vi "C8855-01_CalcuP.vi"(8 "MainD":T1 {"G_DIM" format="%.5f"}, 10 "MP":u32=100 caption="Measurment points" min=1 max=100000, 11 "GT":i32(ring)=4 caption="Gate Time" items=["50 us", "100 us", "200 us", "500 us", "1 ms", "2 ms", "5 ms", "10 ms", "20 ms", "50 ms", "100 ms", "200 ms", "500ms", "1 s", "2 s", "5 s", "10 s"]) -> (0 "MainDR":T1 {"G_DIM" format="%.5f"})   [LabVIEW 2017]
uses:
  C8855_MainD.ctl
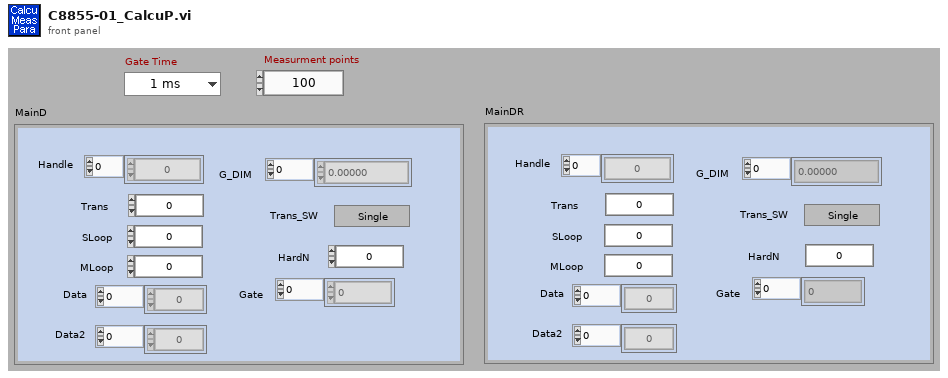
[diagram p1: front panel]
types:
  T1 = typedef "C8855_MainD.ctl" = cluster{"Handle":i64[], "G_DIM":dbl[], "Trans":u16, "Trans_SW":bool, "HardN":i32, "Gate":u8[], "Data":u32[], "Data2":u32[], "SLoop":i32, "MLoop":i32}
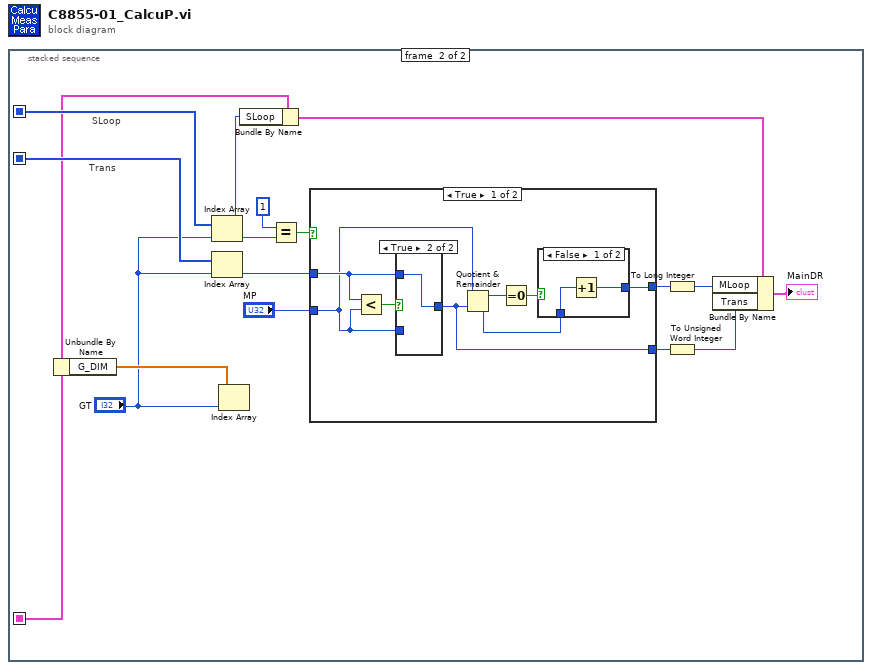
[diagram p0: block diagram]
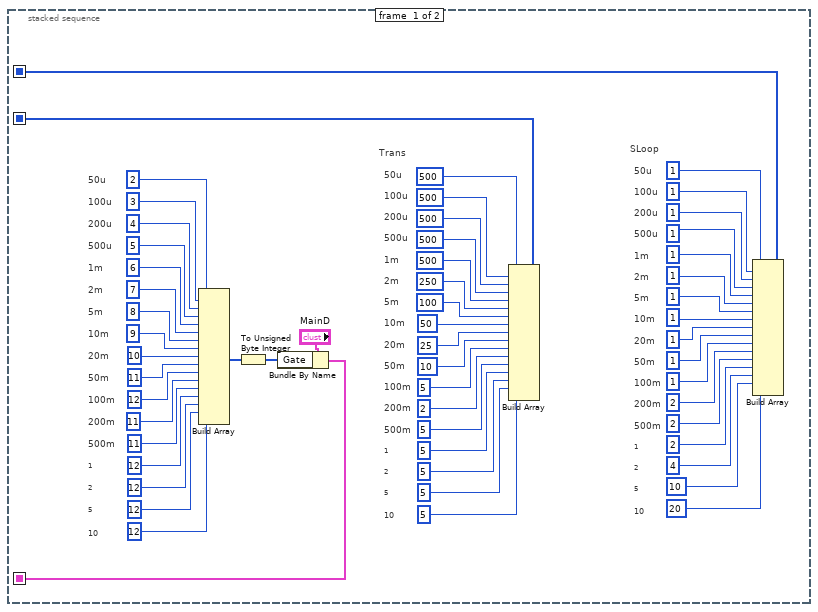
[diagram p2: hidden frame]
diagram:
  n1 = stacked-sequence {
    seq-local: [w1 _] -> [_ w63]
    seq-local: [w5 _] -> [_ w70]
    seq-local: [w4 _] -> [_ w71]
    frame #0 {
      # "10"
      # "5"
      # "2"
      # "1"
      # "500m"
      # "200m"
      # "100m"
      # "50m"
      # "20m"
      # "10m"
      # "5m"
      # "2m"
      # "1m"
      # "500u"
      # "200u"
      # "100u"
      # "50u"
      # "10"
      # "5"
      # "2"
      # "1"
      # "500m"
      # "200m"
      # "100m"
      # "50m"
      # "20m"
      # "10m"
      # "5m"
      # "2m"
      # "1m"
      # "500u"
      # "200u"
      # "100u"
      # "50u"
      # "SLoop"
      # "Trans"
      # "10"
      # "5"
      # "2"
      # "1"
      # "500m"
      # "200m"
      # "100m"
      # "50m"
      # "20m"
      # "10m"
      # "5m"
      # "2m"
      # "1m"
      # "500u"
      # "200u"
      # "100u"
      # "50u"
      n2 = Build Array(2, 3, 4, 5, 6, 7, 8, 9, 10, 11, 12, 11, 11, 12, 12, 12, 12) -> (w23:i32[])
      n3 = To Unsigned Byte Integer(number=w23) -> (unsigned 8bit integer=w2:u8[])
      n4 = Bundle By Name(cluster="MainD", "Gate"=w2) -> (w1:T1)
      n5 = Build Array(u16 500, u16 500, u16 500, u16 500, u16 500, u16 250, u16 100, u16 50, u16 25, u16 10, u16 5, u16 2, u16 5, u16 5, u16 5, u16 5, u16 5) -> (w5:u16[])
      n6 = Build Array(1 ("SLoop"), 1 ("SLoop"), 1 ("SLoop"), 1 ("SLoop"), 1 ("SLoop"), 1 ("SLoop"), 1 ("SLoop"), 1 ("SLoop"), 1 ("SLoop"), 1 ("SLoop"), 1 ("SLoop"), 2 ("SLoop"), 2 ("SLoop"), 2 ("SLoop"), 4 ("SLoop"), 10 ("SLoop"), 20 ("SLoop")) -> (w4:i32[])
    }
    frame #1 {
      # "Trans"
      # "SLoop"
      n7 = Unbundle By Name(w63) -> ("G_DIM"=w72:dbl[])
      n8 = Index Array(array=w71, index="GT") -> (element=w62:i32)
      n9 = Index Array(array=w70, index="GT") -> (element=w65:u16)
      n10 = Index Array(array=w72, index="GT") -> ()  [unwired: 1 out]
      n11 = Bundle By Name(cluster=w63, "SLoop"=w62) -> (w61:T1)
      n12 = Equal?(x=1, y=w62) -> (x = y?=w67:bool)
      n13 = case shown="True" w67 {
        tunnel: [w75 w88] -> w66
        tunnel: w65 -> [w80 w87]
        tunnel: "MP" -> [w79 w88]
        tunnel: [w74 w87] -> w59
        frame True {
          n14 = Less?(x=w80, y=w79) -> (x < y?=w81:bool)
          n15 = case shown="True" w81 {
            tunnel: w79 -> [w85 _]
            tunnel: w80 -> [_ w86]
            tunnel: [w85 w86] -> w74
            frame False {
            }
            frame True {
            }
          }
          n16 = Quotient & Remainder(x=w79, y=w74) -> (x-y*floor(x/y)=w78:u32, floor(x/y)=w76:u32)
          n17 = Equal To 0?(x=w78) -> (x = 0?=w77:bool)
          n18 = case shown="False" w77 {
            tunnel: w76 -> [w83 w84]
            tunnel: [w82 w84] -> w75
            frame False {
              n19 = Increment(x=w83) -> (x+1=w82:u32)
            }
            frame True {
            }
          }
        }
        frame False {
        }
      }
      n20 = To Long Integer(number=w66) -> (32bit integer=w60:i32)
      n21 = To Unsigned Word Integer(number=w59) -> (unsigned 16bit integer=w58:u16)
      n22 = Bundle By Name(cluster=w61, "MLoop"=w60, "Trans"=w58) -> (→"MainDR":T1)
    }
  }
